vi "Init.vi"(11 "Test Case In":refnum<class "Test PCANBasic.lvclass">) -> (0 "error out":errorcluster, 3 "Test Case Out":refnum<class "Test PCANBasic.lvclass">)   [LabVIEW 2020, in "Test PCANBasic.lvclass"]
uses:
  Test PCANBasic.lvclass
  C:/Program Files/National Instruments/LabVIEW 2025/vi.lib/Astemes/LUnit/Test Case.lvclass
  <vilib>/Astemes/LUnit/Test Case.lvclass/Test Case.ctl
  source/PCANBasic.lvlib
  source/PCAN Baud.ctl
  source/TPCANHandle.ctl
  <vilib>/Astemes/LUnit/Test Case.lvclass
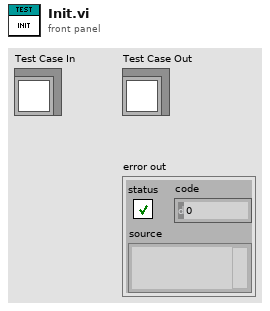
[diagram p1: front panel]
types:
  T1 = typedef "PCANBasic.lvlib/TPCANHandle.ctl" = u16
  T2 = typedef "PCANBasic.lvlib/PCAN Baud.ctl" = u16
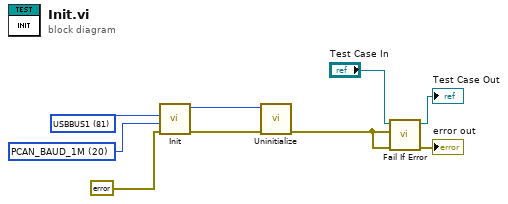
[diagram p0: block diagram]
diagram:
  w4 = T1 81 items=["USBBUS1"=81, "USBBUS2"=82, "USBBUS3"=83, "USBBUS4"=84, "USBBUS5"=85, "USBBUS6"=86, "USBBUS7"=87, "USBBUS8"=88, "USBBUS9"=1289, "USBBUS10"=1290, "USBBUS11"=1291, "USBBUS12"=1292, "USBBUS13"=1293, "USBBUS14"=1294, "USBBUS15"=1295, "USBBUS16"=1296] ("Channel")
  w5 = T2 20 items=["PCAN_BAUD_1M"=20, "PCAN_BAUD_800K"=22, "PCAN_BAUD_500K"=28, "PCAN_BAUD_250K"=284, "PCAN_BAUD_125K"=796, "PCAN_BAUD_100K"=17199, "PCAN_BAUD_95K"=49998, "PCAN_BAUD_83K"=34091, "PCAN_BAUD_50K"=18223, "PCAN_BAUD_47K"=5140, "PCAN_BAUD_33K"=35631, "PCAN_BAUD_20K"=21295, "PCAN_BAUD_10K"=26415, "PCAN_BAUD_5K"=32639] ("Baudrate")
  n1 = call "Init.vi"("error in"=errorcluster {"status"=FALSE, "code"=0, "source"=""}, "Baudrate"=w5, "Channel"=w4) -> ("error out"=w6:errorcluster, "TPCANHandle"=w2:T1)  [unwired: 6 in, 1 out]
  n2 = call "Uninitialize.vi"("error in"=w6, "TPCANHandle"=w2) -> ("error out"=w1:errorcluster)  [unwired: 8 in, 1 out]
  n3 = call <vilib>:"Fail If Error.vi"("error in (no error)"=w1, "Assert error"=w1, "LUnit Test Case In"="Test Case In") -> ("error out"=→"error out":errorcluster, "LUnit Test Case Out"=→"Test Case Out":refnum<class "Test PCANBasic.lvclass">)  [unwired: 7 in]
